vi "Check Parameters.vi"(0 "MRN in":refnum<class "Moving Ripple Noise.lvclass">, 9 "Fs (Hz)":dbl, 11 "error in (no error)":errorcluster) -> (4 "MRN out":refnum<class "Moving Ripple Noise.lvclass">, 15 "error out":errorcluster)   [LabVIEW 2015, in "Moving Ripple Noise.lvclass"]
uses:
  Moving Ripple Noise.lvclass
  Moving Ripple Noise.lvclass/Moving Ripple Noise.ctl
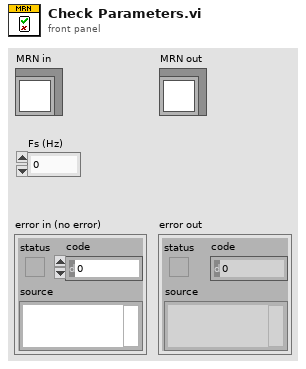
[diagram p1: front panel]
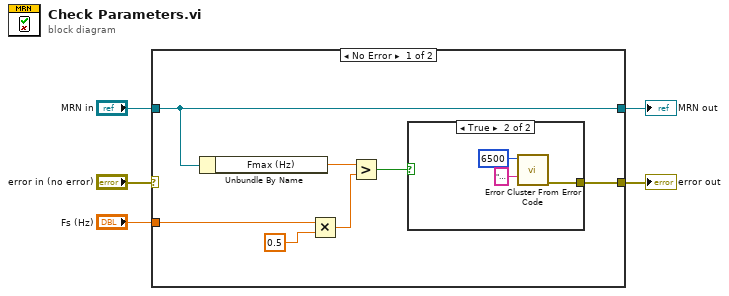
[diagram p0: block diagram]
diagram:
  n1 = case shown="No Error" "error in (no error)" {
    selector: "error in (no error)" -> [_ w17]
    tunnel: [w6 w17] -> w4
    tunnel: [w8 w16] -> w2
    tunnel: "MRN in" -> [w8 w16]
    tunnel: "Fs (Hz)" -> [w7 _]
    frame No Error {
      n2 = Unbundle By Name(w8) -> ("Fmax (Hz)"=w11:dbl)
      n3 = Multiply(x=w7, y=0.5) -> (x*y=w9:dbl)
      n4 = Greater?(x=w11, y=w9) -> (0:w12:bool)
      n5 = case shown="True" w12 {
        tunnel: [_ w14] -> w6
        frame False {
        }
        frame True {
          n6 = call <vilib>:"Error Cluster From Error Code.vi"("error message (\"\")"="Moving Ripple Noise: Fmax exceeds the Nyquist frequency. Increase the sampling rate or decrease Fmax." ("error message (\"\")"), "error code (0)"=6500) -> ("error out"=w14:errorcluster)  [unwired: 7 in]
        }
      }
    }
    frame Error {
    }
  }
  "error out" <- w4
  "MRN out" <- w2
